vi "Band Magnitude - Peak (Orders).vi"(0 "power spectrum [EU^2 rms]":cluster{"f0":dbl, "df":dbl, "magnitude":sgl[]} {"magnitude" format="%.2p"; "df" format="%.2p"; "f0" format="%.2p"}, 1 "Speed (RPM)":sgl, 5 "Start":dbl, 7 "Stop":dbl, 11 "error in (no error)":errorcluster) -> (6 "Max Peak in Band [EU rms]":sgl, 15 "error out":errorcluster)   [LabVIEW 2017, in "VibrationAnalysisFunctions.lvlib"]
uses:
  <vilib>/addons/InsightCM/Utilities/Analysis/Vibration/VibrationAnalysisFunctions.lvlib
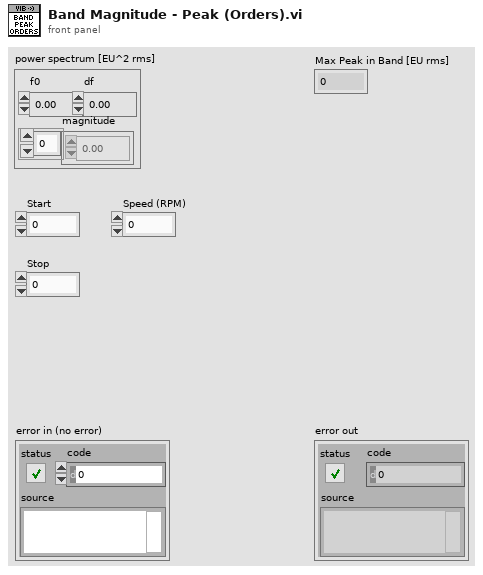
[diagram p1: front panel]
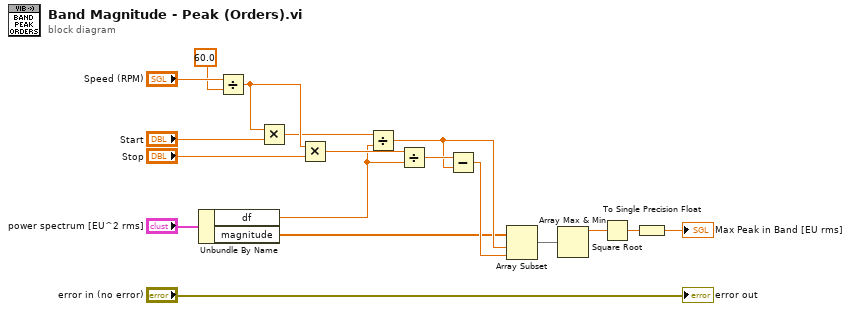
[diagram p0: block diagram]
diagram:
  n1 = Unbundle By Name("power spectrum [EU^2 rms]") -> ("df"=w4:dbl, "magnitude"=w3:sgl[])
  n2 = Divide(x="Speed (RPM)", y=60.0) -> (x/y=w15:dbl)
  n3 = Multiply(x=w15, y="Start") -> (x*y=w6:dbl)
  n4 = Multiply(x=w15, y="Stop") -> (x*y=w5:dbl)
  n5 = Divide(x=w6, y=w4) -> (x/y=w10:dbl)
  n6 = Divide(x=w5, y=w4) -> (x/y=w11:dbl)
  n7 = Subtract(x=w11, y=w10) -> (x-y=w9:dbl)
  n8 = Array Subset(array=w3, index=w10, length=w9) -> (w8:sgl[])
  n9 = Array Max & Min(array=w8) -> (max value=w2:sgl)  [unwired: 3 out]
  n10 = Square Root(x=w2) -> (sqrt(x)=w1:sgl)
  n11 = To Single Precision Float(number=w1) -> (single precision float=→"Max Peak in Band [EU rms]":sgl)
  "error out" <- "error in (no error)"
